vi "Utility MXA-PXA Sweep Complete.vi"(8 "Error In":errorcluster, 9 "Max Time (s)":u32=10000) -> (0 "Error Out":errorcluster, 1 "TimedOut":bool, 2 "Completed":bool, 5 "StatusByte":string)   [LabVIEW 2015]
panel:
  out "VISA Resource Out":refnum<visa-resource-name>
  in  "SA Model":enum16{"PSA", "ESA", "PXA", "MXA"}(ring)
  in  "VISA Resource In":refnum<visa-resource-name>
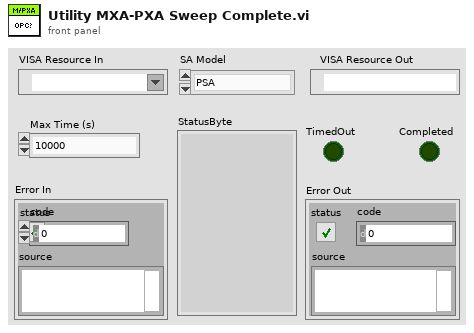
[diagram p1: front panel]
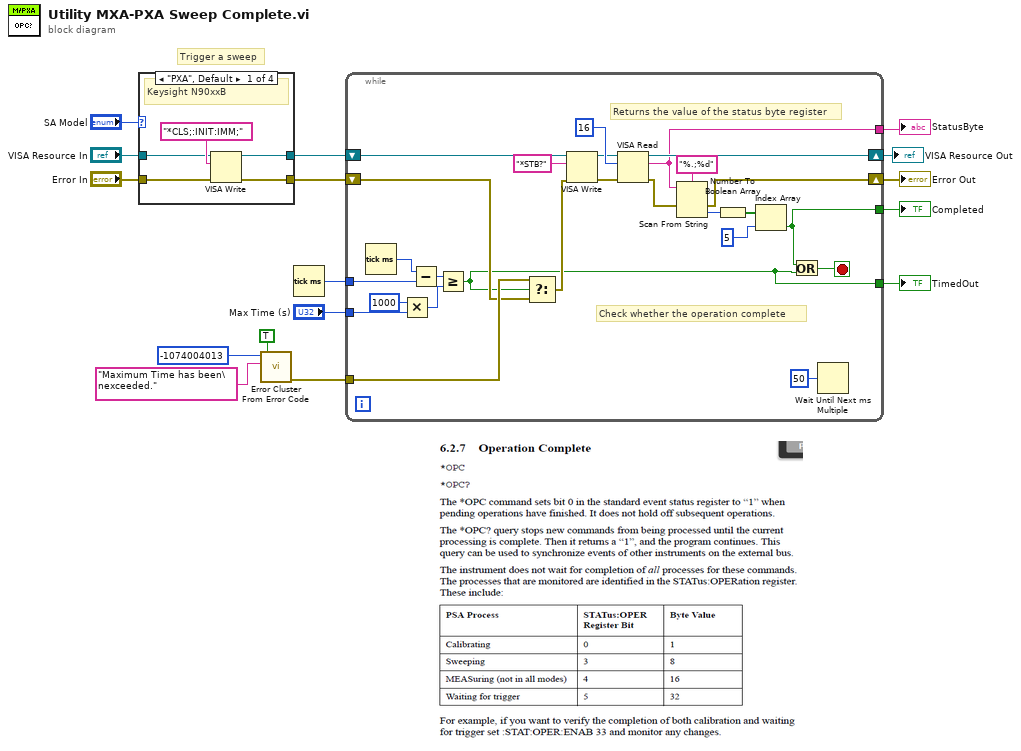
[diagram p0: block diagram]
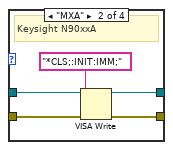
[diagram p2: hidden frame]
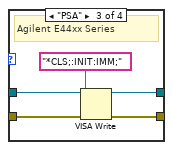
[diagram p3: hidden frame]
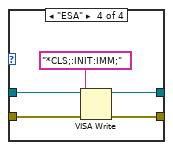
[diagram p4: hidden frame]
diagram:
  # "Trigger a sweep"
  n1 = case shown="\"PXA\", Default" "SA Model" {
    tunnel: [w21 w26 w31 w36] -> w10
    tunnel: [w20 w25 w30 w35] -> w9
    tunnel: "Error In" -> [w18 w24 w29 w34]
    tunnel: "VISA Resource In" -> [w17 w23 w28 w33]
    frame "PXA", Default {
      # "Keysight N90xxB"
      n2 = VISA Write(VISA resource name=w17, write buffer="*CLS;:INIT:IMM;", error in (no error)=w18) -> (VISA resource name out=w21:refnum<visa-resource-name>, error out=w20:errorcluster)  [unwired: 1 out]
    }
    frame "MXA" {
      # "Keysight N90xxA"
      n3 = VISA Write(VISA resource name=w23, write buffer="*CLS;:INIT:IMM;", error in (no error)=w24) -> (VISA resource name out=w26:refnum<visa-resource-name>, error out=w25:errorcluster)  [unwired: 1 out]
    }
    frame "PSA" {
      # "Agilent E44xx Series"
      n4 = VISA Write(VISA resource name=w28, write buffer="*CLS;:INIT:IMM;", error in (no error)=w29) -> (VISA resource name out=w31:refnum<visa-resource-name>, error out=w30:errorcluster)  [unwired: 1 out]
    }
    frame "ESA" {
      n5 = VISA Write(VISA resource name=w33, write buffer="*CLS;:INIT:IMM;", error in (no error)=w34) -> (VISA resource name out=w36:refnum<visa-resource-name>, error out=w35:errorcluster)  [unwired: 1 out]
    }
  }
  n6 = call <vilib>:"Error Cluster From Error Code.vi"("show call chain? (False)"=TRUE, "error message (\"\")"="Maximum Time has been\nexceeded." ("error message (\"\")"), "error code (0)"=-1074004013) -> ("error out"=w11:errorcluster)  [unwired: 6 in]
  n7 = Tick Count (ms)() -> (millisecond timer value=w15:u32)
  n8 = while {
    tunnel: "Max Time (s)" -> [w45]
    tunnel: w15 -> [w54]
    tunnel: w11 -> [w42]
    shift-right: [w44] -> w8
    shift-left: w9 -> [w41]
    shift-right: [w61] -> w1
    shift-left: w10 -> [w58]
    tunnel: [w43] -> w7
    tunnel: [w40] -> w6
    tunnel: [w39] -> w5
    stop <- w49 stop-if-true
    # "Check whether the operation complete"
    # "Returns the value of the status byte register"
    n9 = Tick Count (ms)() -> (millisecond timer value=w55:u32)
    n10 = Multiply(x=u32 1000, y=w45) -> (x*y=w38:u32)
    n11 = Subtract(x=w55, y=w54) -> (x-y=w46:u32)
    n12 = Greater Or Equal?(x=w46, y=w38) -> (x >= y?=w40:bool)
    n13 = Select(t=w42, s=w40, f=w41) -> (s? t:f=w48:errorcluster)
    n14 = VISA Write(VISA resource name=w58, write buffer="*STB?", error in (no error)=w48) -> (VISA resource name out=w56:refnum<visa-resource-name>, error out=w57:errorcluster)  [unwired: 1 out]
    n15 = VISA Read(VISA resource name=w56, byte count=u32 16, error in (no error)=w57) -> (VISA resource name out=w61:refnum<visa-resource-name>, read buffer=w39:string, error out=w53:errorcluster)  [unwired: 1 out]
    n16 = Scan From String(format string="%.;%d", input string=w39, error in=w53) -> (error out=w44:errorcluster, output 1=w50:i32)  [unwired: 2 in, 2 out]
    n17 = Number To Boolean Array(number=w50) -> (Boolean array=w51:bool[])
    n18 = Index Array(array=w51, index=5) -> (element=w43:bool)
    n19 = Or(x=w43, y=w40) -> (x .or. y?=w49:bool)
    n20 = Wait Until Next ms Multiple(millisecond multiple=u32 50 ("milliseconds to wait")) -> ()  [unwired: 1 out]
  }
  "Error Out" <- w8
  "Completed" <- w7
  "TimedOut" <- w6
  "StatusByte" <- w5
  "VISA Resource Out" <- w1
